vi "Generate Arguments.vi"(7 "is subsystem":bool, 8 "error in (no error)":errorcluster, 9 "command":string, 11 "client in":refnum<class "Direct SFTP Connection.lvclass">) -> (0 "error out":errorcluster, 2 "arguments":string[](array[string]), 3 "client out":refnum<class "Direct SFTP Connection.lvclass">, 5 "environment variables":cluster{"name":string, "value":string}[](array[cluster]))   [LabVIEW 2020, in "NI_SFTP.lvlib" / "Direct SFTP Connection.lvclass"]
uses:
  <vilib>/net/SFTP/Direct SFTP Connection/Direct SFTP Connection.lvclass
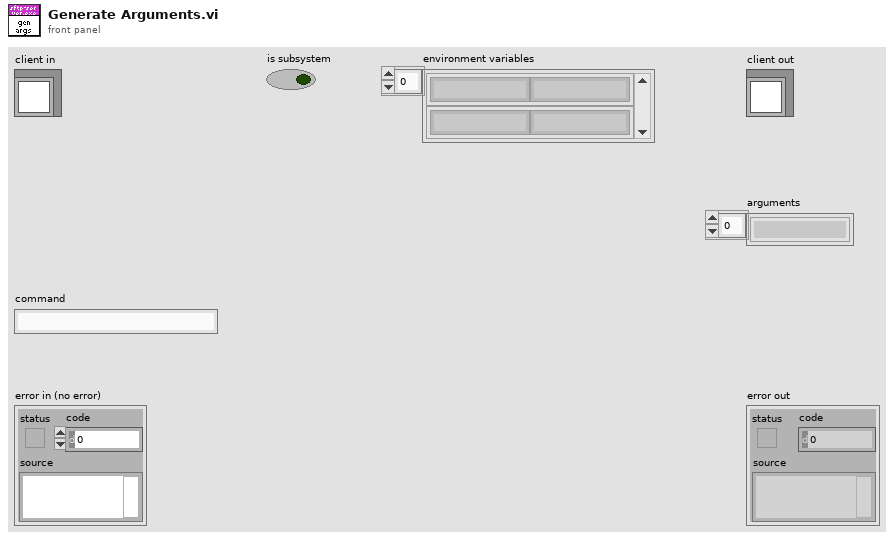
[diagram p1: front panel]
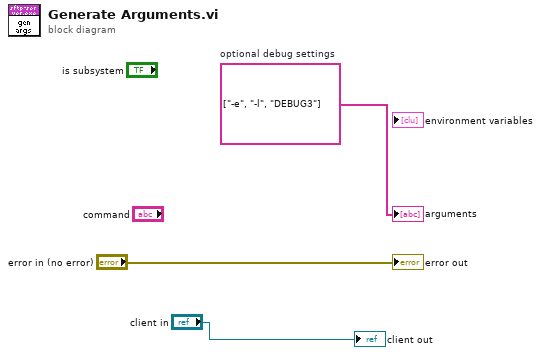
[diagram p0: block diagram]
diagram:
  w3 = string[] ["-e", "-l", "DEBUG3"]  # optional debug settings
  "error out" <- "error in (no error)"
  "client out" <- "client in"
  "arguments" <- w3
